vi "Subvi_Training_LDA.vi"(0 "Input_Data":dbl[][](array[numeric])) -> (1 "A * B 2":T1 caption="A * B(Point)", 2 "A * B":T1 caption="A * B(Matrix)")   [LabVIEW 2014]
uses:
  <vilib>/Analysis/Matrix/Datatypes/RealMatrix.ctl
  <vilib>/Analysis/baseanly.llb/Mean (DBL).vi
  <vilib>/Analysis/baseanly.llb/Real A x B.vi
  <vilib>/Analysis/7linalg.llb/Real Transpose Matrix.vi
  <vilib>/Analysis/Matrix/Numeric/Conversions/Array To Matrix - RA2.vi
  <vilib>/Analysis/Matrix/Numeric/Multiply/Multiply - RM,R.vi
  <vilib>/Analysis/Matrix/Numeric/Add/Add - RM,RM.vi
  <vilib>/Analysis/baseanly.llb/Real Inverse Matrix.vi
  <vilib>/Analysis/Matrix/Numeric/Conversions/Array To Matrix - RA.vi
  <vilib>/Analysis/Matrix/Numeric/Subtract/Subtract - RM,RM.vi
  <vilib>/Analysis/Matrix/Numeric/Multiply/Multiply - R,RM.vi
  <vilib>/Analysis/Matrix/Numeric/Multiply/Multiply - RM,RM.vi
  <vilib>/Analysis/Matrix/NI_Matrix.lvlib
  <vilib>/Analysis/NI_AALBase.lvlib
  <vilib>/Analysis/NI_AALPro.lvlib
panel:
  out "size(s) 2":i32[](array[numeric])
  out "size(s)":i32[](array[numeric])
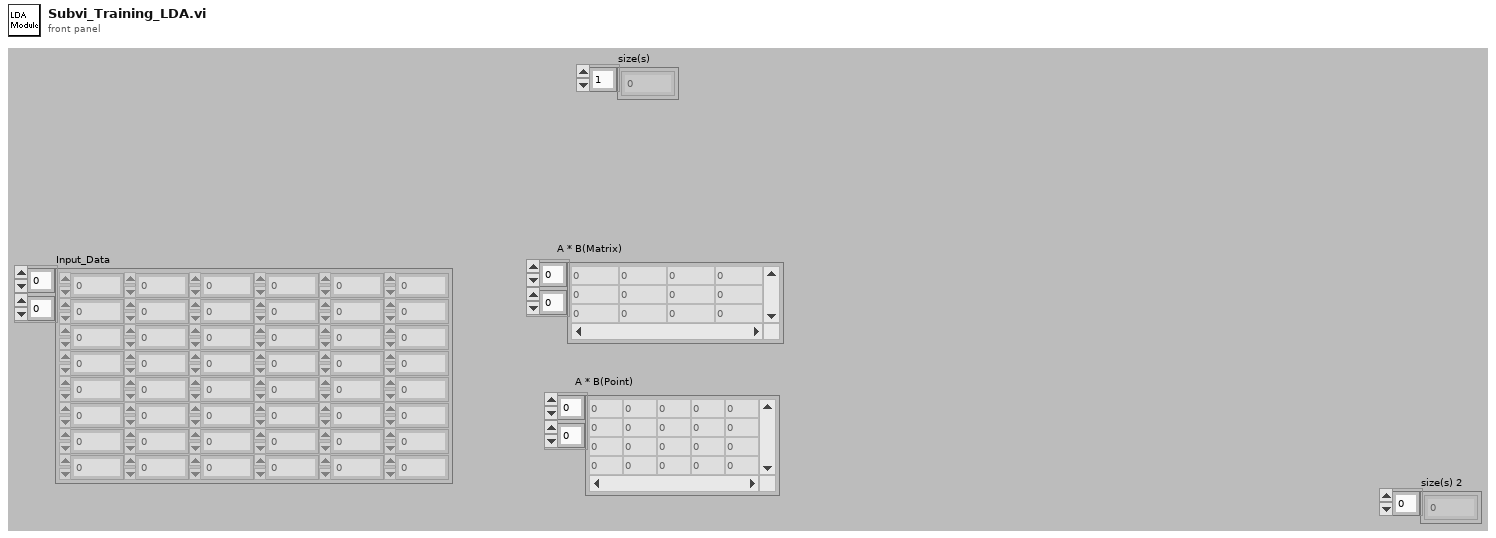
[diagram p1: front panel]
types:
  T1 = typedef "NI_Matrix.lvlib/RealMatrix.ctl" = dbl[][]
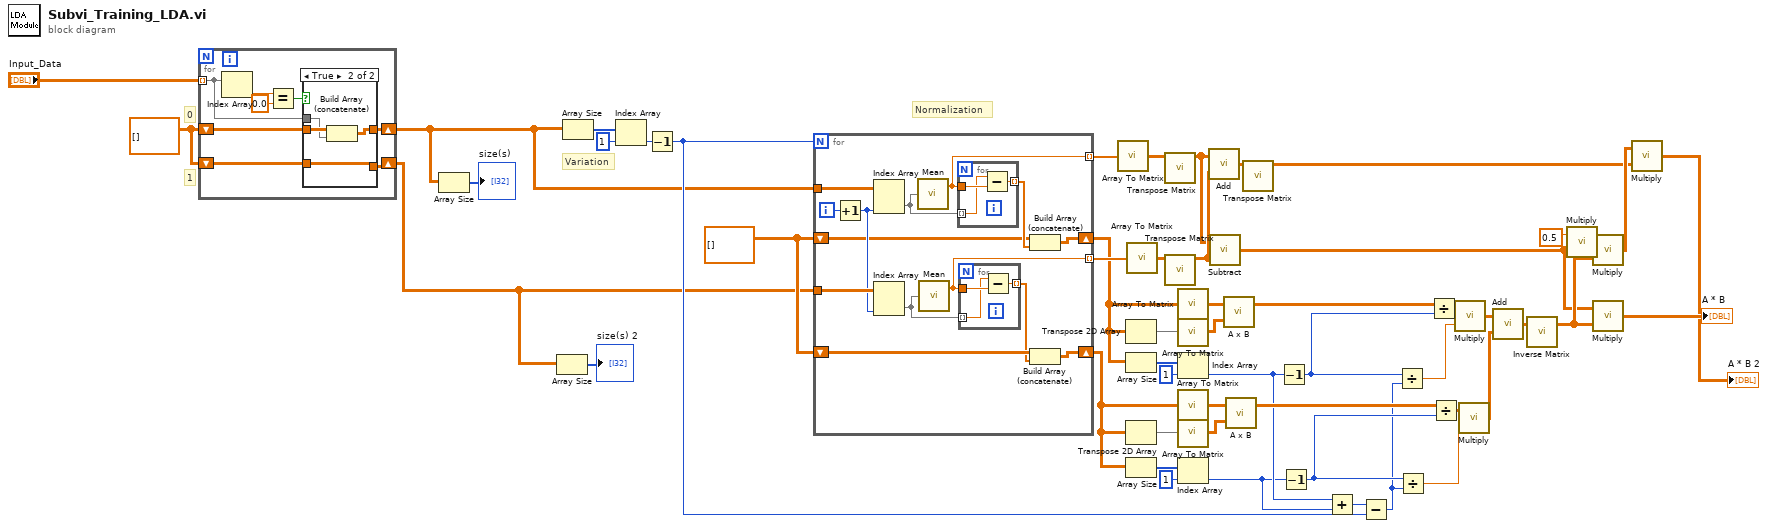
[diagram p0: block diagram]
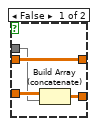
[diagram p2: hidden frame]
diagram:
  w49 = dbl[][] []
  w53 = dbl[][] []
  # "Normalization"
  # "Variation"
  # "1"
  # "0"
  n1 = for {
    tunnel: "Input_Data" -> [w58] mode=indexing
    shift-right: [w55] -> w4
    shift-left: w53 -> [w57]
    shift-right: [w54] -> w1
    shift-left: w53 -> [w56]
    n2 = Index Array(array=w58) -> (element=w61:dbl)  [unwired: 1 in]
    n3 = Equal?(x=w61, y=0.0) -> (x = y?=w59:bool)
    n4 = case shown="True" w59 {
      tunnel: w58 -> [w62 w68]
      tunnel: w57 -> [w65 w69]
      tunnel: w56 -> [w64 w66]
      tunnel: [w65 w67] -> w55
      tunnel: [w63 w66] -> w54
      frame False {
        n5 = Build Array (concatenate)(w64, w62) -> (w63:dbl[][])
      }
      frame True {
        n6 = Build Array (concatenate)(w69, w68) -> (w67:dbl[][])
      }
    }
  }
  n7 = Array Size(array=w4) -> (size(s)=→"size(s)":i32[])
  n8 = Array Size(array=w1) -> (size(s)=→"size(s) 2":i32[])
  n9 = Array Size(array=w4) -> (size(s)=w52:i32[])
  n10 = Index Array(array=w52, index=1) -> (element=w50:i32)
  n11 = Decrement(x=w50) -> (x-1=w24:i32)
  n12 = for {
    N: w24 -> [_]
    tunnel: w1 -> [w82]
    tunnel: w4 -> [w83]
    shift-right: [w76] -> w36
    shift-left: w49 -> [w75]
    shift-right: [w73] -> w34
    shift-left: w49 -> [w74]
    tunnel: [w71] -> w48 mode=indexing
    tunnel: [w70] -> w47 mode=indexing
    i -> [w81]
    n13 = Increment(x=w81) -> (x+1=w80:i32)
    n14 = Index Array(array=w83, index (col)=w80) -> (element=w79:dbl[])  [unwired: 1 in]
    n15 = Index Array(array=w82, index (col)=w80) -> (element=w78:dbl[])  [unwired: 1 in]
    n16 = call-poly <vilib>:"Mean.vi"("X"=w79) -> ("mean"=w71:dbl)  [unwired: 1 out]
    n17 = call-poly <vilib>:"Mean.vi"("X"=w78) -> ("mean"=w70:dbl)  [unwired: 1 out]
    n18 = for {
      tunnel: w71 -> [w89]
      tunnel: w79 -> [w88] mode=indexing
      tunnel: [w87] -> w77 mode=indexing
      n19 = Subtract(x=w88, y=w89) -> (x-y=w87:dbl)
    }
    n20 = for {
      tunnel: w70 -> [w86]
      tunnel: w78 -> [w85] mode=indexing
      tunnel: [w84] -> w72 mode=indexing
      n21 = Subtract(x=w85, y=w86) -> (x-y=w84:dbl)
    }
    n22 = Build Array (concatenate)(w75, w77) -> (w76:dbl[][])
    n23 = Build Array (concatenate)(w74, w72) -> (w73:dbl[][])
  }
  n24 = call-poly <vilib>:"Array To Matrix.vi"("Real 1D Array"=w48) -> ("Real Matrix (Column Vector)"=w46:T1)
  n25 = Transpose 2D Array(2D array=w36) -> (transposed array=w37:dbl[][])
  n26 = Array Size(array=w36) -> (size(s)=w38:i32[])
  n27 = Transpose 2D Array(2D array=w34) -> (transposed array=w35:dbl[][])
  n28 = Array Size(array=w34) -> (size(s)=w41:i32[])
  n29 = call-poly <vilib>:"Array To Matrix.vi"("Real 1D Array"=w47) -> ("Real Matrix (Column Vector)"=w45:T1)
  n30 = call-poly <vilib>:"Transpose Matrix.vi"("Input Matrix"=w46) -> ("Matrix Transpose"=w43:T1)  [unwired: 9 in, 1 out]
  n31 = call-poly <vilib>:"Transpose Matrix.vi"("Input Matrix"=w45) -> ("Matrix Transpose"=w44:T1)  [unwired: 9 in, 1 out]
  n32 = call-poly <vilib>:"Array To Matrix.vi"("Real 2D Array"=w36) -> ("Real Matrix"=w33:T1)
  n33 = call-poly <vilib>:"Array To Matrix.vi"("Real 2D Array"=w37) -> ("Real Matrix"=w32:T1)
  n34 = Index Array(array=w38, index=1) -> (element=w27:i32)
  n35 = call-poly <vilib>:"Array To Matrix.vi"("Real 2D Array"=w34) -> ("Real Matrix"=w31:T1)
  n36 = call-poly <vilib>:"Array To Matrix.vi"("Real 2D Array"=w35) -> ("Real Matrix"=w30:T1)
  n37 = Index Array(array=w41, index=1) -> (element=w26:i32)
  n38 = call-poly <vilib>:"Add.vi"("Real Matrix B"=w44, "Real Matrix A"=w43) -> ("A + B"=w42:T1)
  n39 = call-poly <vilib>:"Subtract.vi"("Real Matrix B"=w44, "Real Matrix A"=w43) -> ("A - B"=w6:T1)
  n40 = call-poly <vilib>:"A x B.vi"("B"=w32, "A"=w33) -> ("A x B"=w29:T1)  [unwired: 1 out]
  n41 = call-poly <vilib>:"A x B.vi"("B"=w30, "A"=w31) -> ("A x B"=w28:T1)  [unwired: 1 out]
  n42 = call-poly <vilib>:"Transpose Matrix.vi"("Input Matrix"=w42) -> ("Matrix Transpose"=w7:T1)  [unwired: 9 in, 1 out]
  n43 = Decrement(x=w27) -> (x-1=w23:i32)
  n44 = Decrement(x=w26) -> (x-1=w22:i32)
  n45 = Add(x=w27, y=w26) -> (x+y=w25:i32)
  n46 = Subtract(x=w25, y=w24) -> (x-y=w21:i32)
  n47 = Divide(x=w23, y=w21) -> (x/y=w19:dbl)
  n48 = Divide(x=w22, y=w21) -> (x/y=w17:dbl)
  n49 = Divide(x=w29, y=w23) -> (x/y=w20:T1)
  n50 = Divide(x=w28, y=w22) -> (x/y=w18:T1)
  n51 = call-poly <vilib>:"Multiply.vi"("Real Scalar c"=w19, "Real Matrix A"=w20) -> ("A * c"=w16:T1)
  n52 = call-poly <vilib>:"Multiply.vi"("Real Scalar c"=w17, "Real Matrix A"=w18) -> ("A * c"=w15:T1)
  n53 = call-poly <vilib>:"Add.vi"("Real Matrix B"=w15, "Real Matrix A"=w16) -> ("A + B"=w14:T1)
  n54 = call-poly <vilib>:"Inverse Matrix.vi"("Input Matrix"=w14) -> ("Inverse Matrix"=w11:T1)  [unwired: 1 in, 1 out]
  n55 = call-poly <vilib>:"Multiply.vi"("Real Matrix A"=w6, "Real Scalar c"=0.5) -> ("c * A"=w12:T1)
  n56 = call-poly <vilib>:"Multiply.vi"("Real Matrix B"=w11, "Real Matrix A"=w12) -> ("A * B"=w10:T1)
  n57 = call-poly <vilib>:"Multiply.vi"("Real Matrix B"=w11, "Real Matrix A"=w6) -> ("A * B"=→"A * B":T1)
  n58 = call-poly <vilib>:"Multiply.vi"("Real Matrix B"=w7, "Real Matrix A"=w10) -> ("A * B"=→"A * B 2":T1)
